vi "Config Observation Time.vi"(0 "VISA resource name":refnum<visa-resource-name>, 5 "Observation Time (12: 100msec)":u16(ring)=12 items=["1ksec", "400sec", "200sec", "100sec", "40sec", "20sec", "10sec", "4sec", "2sec", "1sec", "400msec", "200msec", "100msec", "40msec", "20msec", "10msec", "4msec", "2msec", "1msec", "400usec", "200usec", "100usec", "40usec", "20usec", "10usec"], 11 "error in (no error)":errorcluster) -> (4 "VISA resource name out":refnum<visa-resource-name>, 15 "error out":errorcluster)   [LabVIEW 2013, in "Yokogawa PZ4000.lvlib"]
doc: "This VI sends the Observation Time command to the PZ4000 series."
uses:
  Yokogawa PZ4000.lvlib
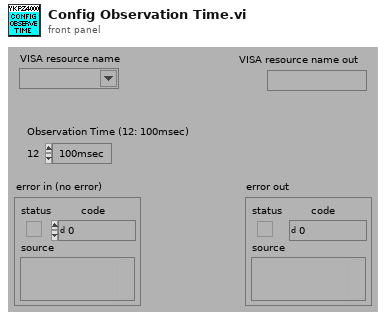
[diagram p1: front panel]
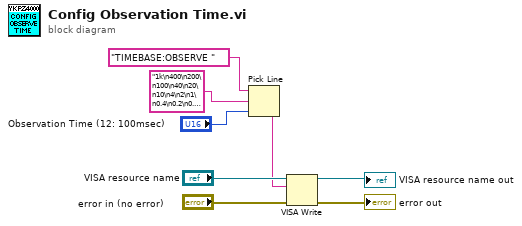
[diagram p0: block diagram]
diagram:
  n1 = Pick Line(string ("")="TIMEBASE:OBSERVE ", multi-line string="1k\n400\n200\n100\n40\n20\n10\n4\n2\n1\n0.4\n0.2\n0.1\n0.04\n0.02\n0.01\n0.004\n0.002\n0.001\n0.0004\n0.0002\n0.0001", line index="Observation Time (12: 100msec)") -> (output string=w3:string)
  n2 = VISA Write(VISA resource name="VISA resource name", write buffer=w3, error in (no error)="error in (no error)") -> (VISA resource name out=→"VISA resource name out":refnum<visa-resource-name>, error out=→"error out":errorcluster)  [unwired: 1 out]
